vi "Tetra_Read UCD.vi"(0 "COMPORT":refnum<visa-resource-name>="COM4", 11 "error in (no error)":errorcluster, 12 "Open Ser(t)":bool, 13 "Clear errors in(t)":bool, 14 "Close Ser(t)":bool) -> (3 "rdv":dbl[](array[numeric]), 4 "comport":refnum<visa-resource-name>="COM4", 15 "error out":errorcluster)   [LabVIEW 2018]
panel:
  out "Names":string[](array[string])
  out "Rdv":string
  # "rdiv\n0)  sw3p6:   186 mA  3600 mV\n1)  sw5p5:    89 mA  5496 mV\n2) sw2p8a:   321 mA  2776 mV\n3) sw2p8b:   334 mA  2768 mV\n4)  sw2p4:  1481 mA  2280 mV\n5)  sw1p4:   556 mA  1360 mV\n>"
  # "0)  isu18p5\n1)  core1p0\n2)   xvr1p0\n3)   dig1p8\n4)   dig3p3\n5)   xvr1p2\n6)   div5p0\n7)   vdd3p3\n8)    rx2p5\n9)    tx2p5"
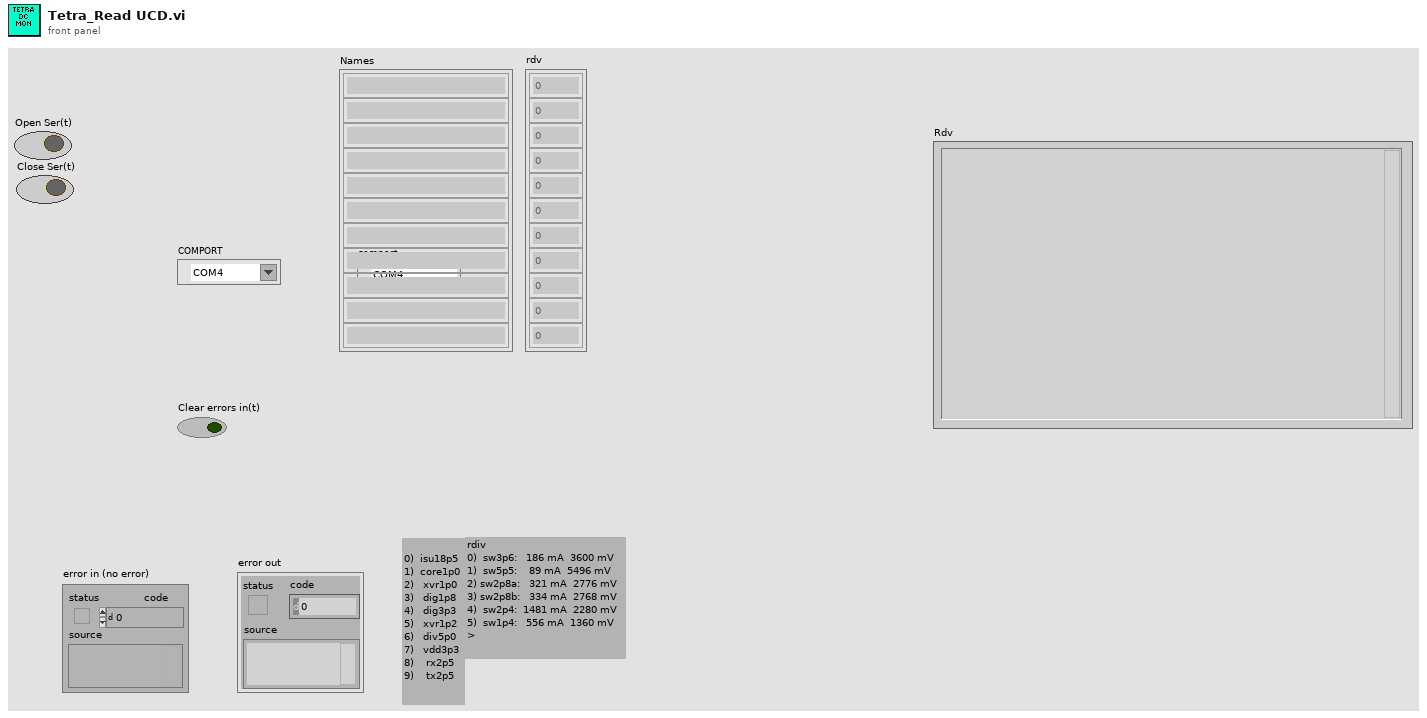
[diagram p1: front panel]
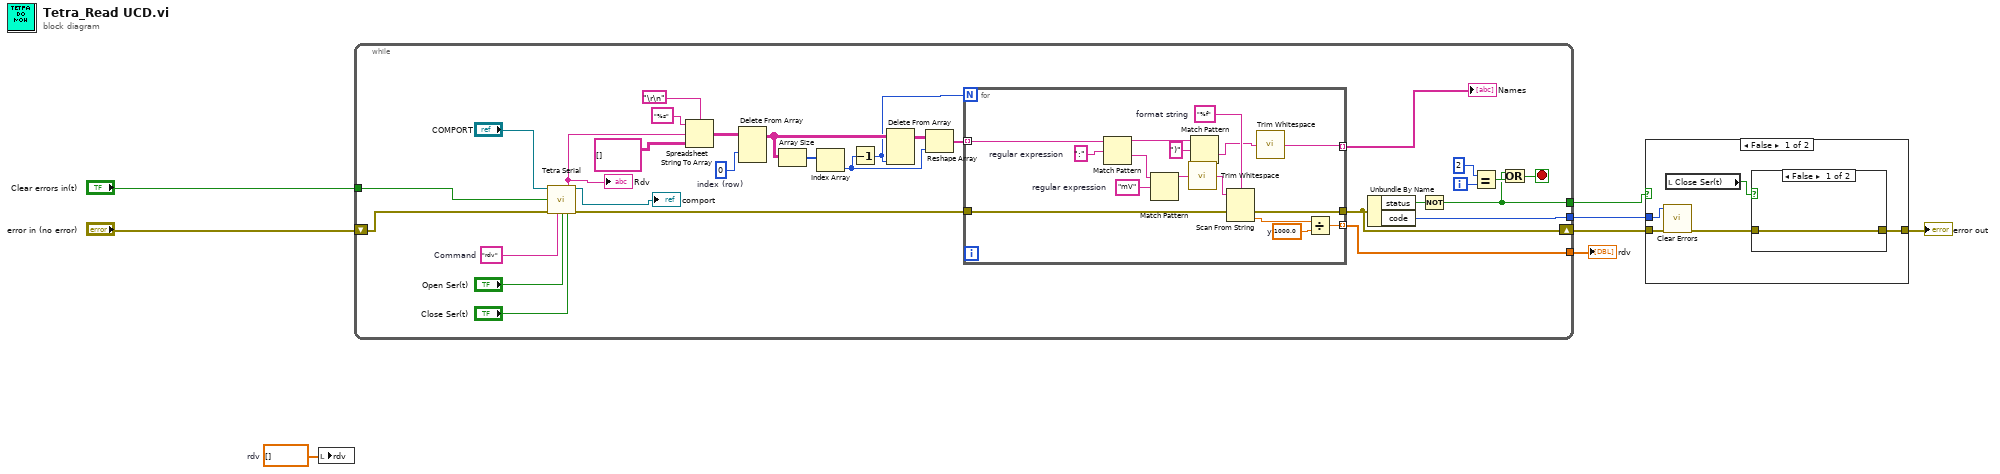
[diagram p0: block diagram]
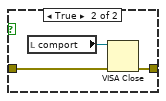
[diagram p2: hidden frame]
diagram:
  w5 = dbl[] []  # rdv
  n1 = local write "rdv"(w5) -> ()
  n2 = while {
    tunnel: [w38] -> w8
    tunnel: "Clear errors in(t)" -> [w9]
    shift-right: [w26] -> w3
    shift-left: "error in (no error)" -> [w10]
    tunnel: [w20] -> w4
    tunnel: [w19] -> w1
    i -> [w22]
    stop <- w25 stop-if-true
    w27 = "rdv"  # Command
    w34 = 0  # index (row)
    n3 = call "Tetra Serial.vi"("COMPORT"="COMPORT", "ClearErrorIn(t)"=w9, "error in (no error)"=w10, "Command"=w27, "Open Ser(t)"="Open Ser(t)", "Close Ser(t)"="Close Ser(t)") -> ("output"=w30:string, "comport"=→"comport":refnum<visa-resource-name>, "error out"=w28:errorcluster)  [unwired: 5 in, 2 out]
    "Rdv" <- w30
    n4 = Spreadsheet String To Array(delimiter (Tab)="\r\n", format string="%s", spreadsheet string=w30, array type (2D Dbl)=string[][] []) -> (array=w16:string[][])
    n5 = Delete From Array(array=w16, index (row)=w34) -> (array with subset deleted=w15:string[][])  [unwired: 2 in, 1 out]
    n6 = Array Size(array=w15) -> (size(s)=w14:i32[])
    n7 = Index Array(array=w14) -> (element=w13:i32)  [unwired: 1 in]
    n8 = Decrement(x=w13) -> (x-1=w12:i32)
    n9 = Delete From Array(array=w15, index (col)=w12) -> (array with subset deleted=w33:string[][])  [unwired: 2 in, 1 out]
    n10 = Reshape Array(w33, w13) -> (w32:string[])
    n11 = for {
      N: w12 -> [_]
      tunnel: w32 -> [w54] mode=indexing
      tunnel: [w47] -> w38 mode=indexing
      tunnel: [w44] -> w26
      tunnel: w28 -> [w43]
      tunnel: [w39] -> w11 mode=indexing
      w45 = "%f"  # format string
      w46 = 1000.0  # y
      w51 = "mV"  # regular expression
      w53 = ":"  # regular expression
      n12 = Match Pattern(string=w54, regular expression=w53) -> (before substring=w42:string, after substring=w52:string)  [unwired: 1 in, 2 out]
      n13 = Match Pattern(string=w52, regular expression=w51) -> (before substring=w50:string)  [unwired: 1 in, 3 out]
      n14 = call <vilib>:"Trim Whitespace.vi"("string"=w50) -> ("trimmed string"=w49:string)  [unwired: 1 in]
      n15 = Match Pattern(string=w42, regular expression=")") -> (after substring=w40:string)  [unwired: 1 in, 3 out]
      n16 = Scan From String(format string=w45, input string=w49, error in=w43) -> (error out=w44:errorcluster, output 1=w48:dbl)  [unwired: 2 in, 2 out]
      n17 = call <vilib>:"Trim Whitespace.vi"("string"=w40) -> ("trimmed string"=w39:string)  [unwired: 1 in]
      n18 = Divide(x=w48, y=w46) -> (x/y=w47:dbl)
    }
    "Names" <- w11
    n19 = Unbundle By Name(w26) -> ("status"=w24:bool, "code"=w20:i32)
    n20 = Not(x=w24) -> (.not. x?=w19:bool)
    n21 = Equal?(x=2, y=w22) -> (x = y?=w23:bool)
    n22 = Or(x=w19, y=w23) -> (x .or. y?=w25:bool)
  }
  "rdv" <- w8
  n23 = case shown="False" w1 {
    tunnel: w4 -> [w59 _]
    tunnel: w3 -> [w57 w64]
    tunnel: [w56 w64] -> w2
    frame False {
      n24 = call <vilib>:"Clear Errors.vi"("error in (no error)"=w57, "specific error code to clear (0: all)"=w59) -> ("error out"=w58:errorcluster)  [unwired: 4 in, 1 out]
      n25 = local read "Close Ser(t)"() -> (w55:bool)
      n26 = case shown="False" w55 {
        tunnel: w58 -> [w60 w62]
        tunnel: [w60 w61] -> w56
        frame False {
        }
        frame True {
          n27 = local read "comport"() -> (w63:refnum<visa-resource-name>)
          n28 = VISA Close(VISA resource name=w63, error in (no error)=w62) -> (error out=w61:errorcluster)
        }
      }
    }
    frame True {
    }
  }
  "error out" <- w2
